vi "Init.vi"(8 "error in (no error)":errorcluster, 10 "Shutdown Event":refnum<user-event>, 11 "DAQmx in":refnum<class "DAQmx.lvclass">) -> (0 "error out":errorcluster, 3 "DAQmx out":refnum<class "DAQmx.lvclass">)   [LabVIEW 2019, in "DAQmx.lvlib" / "DAQmx.lvclass"]
uses:
  DAQmx.lvclass
  Plugin Interfaces/Controller Interface/Controller Interface.lvlibp/Controller Interface Class/Controller Interface.lvclass
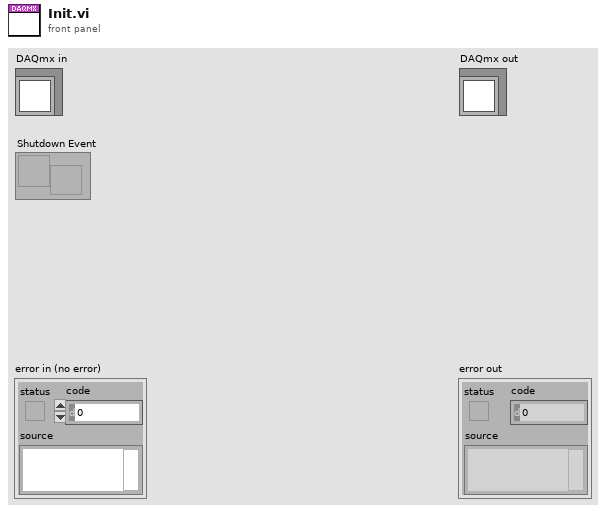
[diagram p1: front panel]
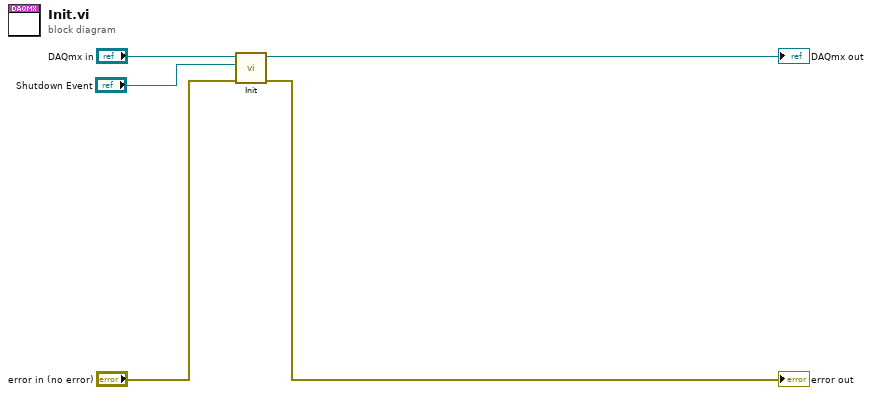
[diagram p0: block diagram]
diagram:
  n1 = call-parent "Init.vi"("error in (no error)"="error in (no error)", "Shuwdown Event"="Shutdown Event", "Controller Interface in"="DAQmx in") -> ("error out"=→"error out":errorcluster, "Controller Interface out"=→"DAQmx out":refnum<class "DAQmx.lvclass">)  [unwired: 7 in]
